vi "PVCAM_SetParam.vi"(8 "error in (no error)":errorcluster, 9 "param_value":u16, 10 "param_id":u32, 11 "hCam":i16) -> (0 "error out":errorcluster, 2 "return type":i16)   [LabVIEW 2021]
uses:
  pvcam64.dll
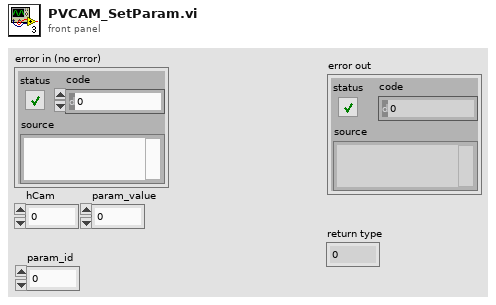
[diagram p1: front panel]
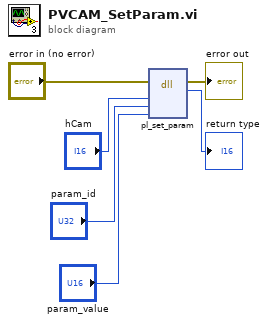
[diagram p0: block diagram]
diagram:
  n1 = dll-call lib="pvcam64.dll" fn="pl_set_param"(error in="error in (no error)", "hCam"="hCam", "param_id"="param_id", "param_value"="param_value") -> (error out=→"error out":errorcluster, "return type"=→"return type":i16)  [unwired: 5 in, 1 out]
